vi "_Untitled 4 (SubVI).vi"(8 "Interpolation factor (n)":i32=2, 9 "Частота, Гц":dbl, 10 "all rows":string[][](array[string])=[["", "50000", "100000", "200000"], ["100", "0", "0", "0"], ["75.3", "-11.3", "-21.7", "-46.55"], ["55.3", "-19.9", "-30.2", "-69.65"], ["35.3", "-30", "-47.2", "-109.2"], ["", "", "", ""], ["", "", "", ""], ["", "", "", ""]], 11 "XYGraph in":refnum<vi>) -> (2 "ArrayFreqOut":dbl[](array[numeric]), 3 "ArrayOut":cluster{dbl[], dbl[]}[](array[cluster]))   [LabVIEW 2017]
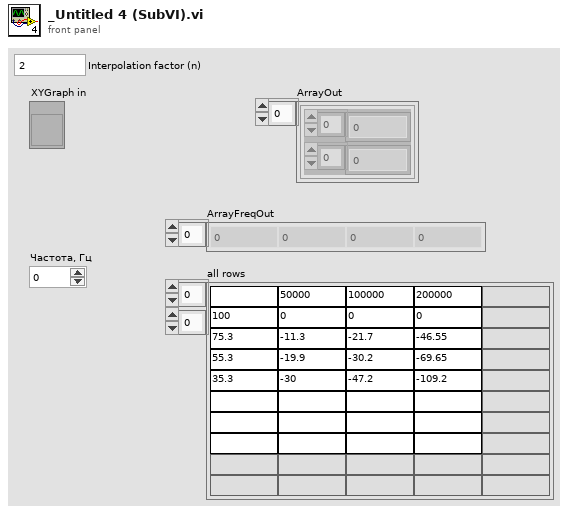
[diagram p1: front panel]
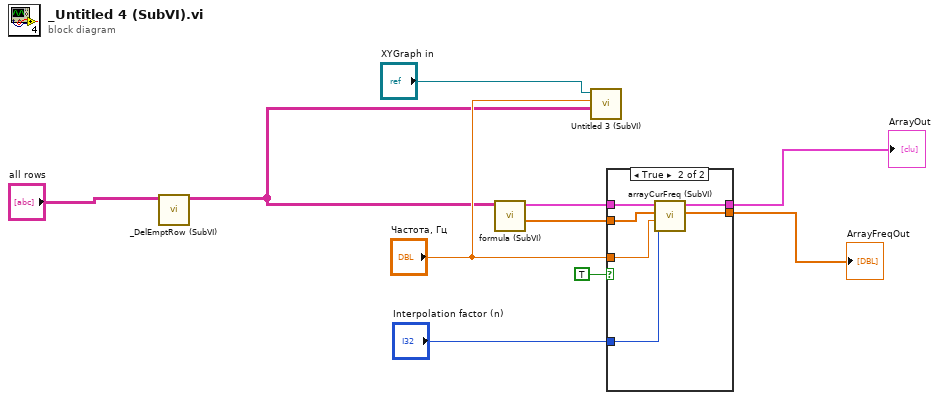
[diagram p0: block diagram]
diagram:
  n1 = call "_DelEmptRow (SubVI).vi"("all rows in"="all rows") -> ("all rows out"=w2:string[][])  [unwired: 10 in]
  n2 = call "formula (SubVI).vi"("Table 2"=w2) -> ("ArrayFreq"=w5:dbl[], "Array 2"=w6:cluster{"X Values":dbl[], "Y Values":dbl[]}[])  [unwired: 9 in]
  n3 = call "Untitled 3 (SubVI).vi"("all rows"=w2, "Частота, Гц"="Частота, Гц", "XYGraph in"="XYGraph in") -> ()  [unwired: 9 in]
  n4 = case shown="True" TRUE {
    tunnel: [w11 w18] -> w10
    tunnel: [w12 w17] -> w9
    tunnel: "Частота, Гц" -> [_ w16]
    tunnel: w6 -> [w12 w15]
    tunnel: w5 -> [w11 w14]
    tunnel: "Interpolation factor (n)" -> [_ w13]
    frame False {
    }
    frame True {
      n5 = call "arrayCurFreq (SubVI).vi"("Interpolation factor (n)"=w13, "Частота, Гц"=w16, "ArrayFreq"=w14, "ArrayIn"=w15) -> ("ArrayFreqOut"=w18:dbl[], "ArrayOut"=w17:cluster{dbl[], dbl[]}[])  [unwired: 6 in]
    }
  }
  "ArrayFreqOut" <- w10
  "ArrayOut" <- w9
